vi "Set LCD to first pixel.vi"(8 "error in":errorcluster, 11 "FPGA VI Reference In":T1) -> (0 "error out":errorcluster, 3 "FPGA VI Reference Out":T1)   [LabVIEW 2019]
uses:
  TypeDefs/FPGA Reference.ctl
  <vilib>/Utility/error.llb/Error Cluster From Error Code.vi
  <vilib>/rvi/errors/niLvFpgaAdjustHostInterfaceError.vi
  <vilib>/rvi/interface/nirviReadWriteControl/nirviReadWriteControl.xnode
  FPGA Bitfiles/adafruitlcdsom_FPGATarget_FPGAMain_K7l+4zj6vFY.lvbitx
  FPGA Main.vi
  NiFpgaLv.dll
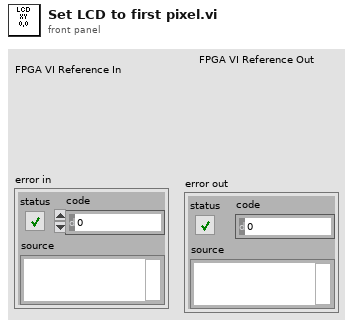
[diagram p1: front panel]
types:
  T1 = typedef "FPGA Reference.ctl" = refnum<k20>
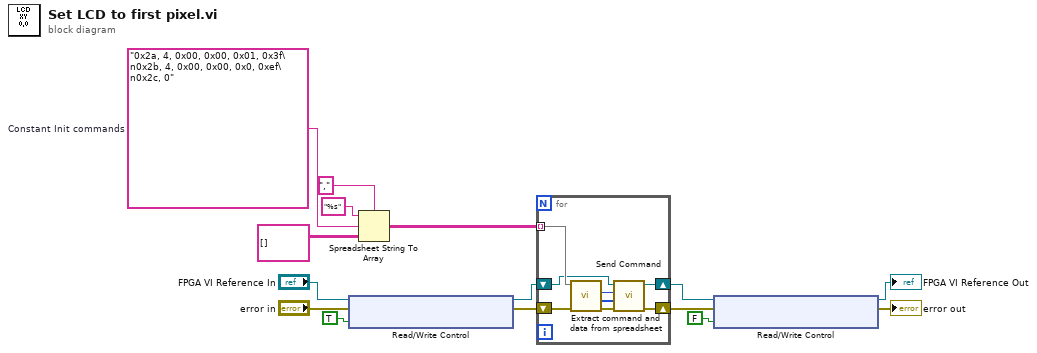
[diagram p0: block diagram]
diagram:
  w3 = "0x2a, 4, 0x00, 0x00, 0x01, 0x3f\n0x2b, 4, 0x00, 0x00, 0x0, 0xef\n0x2c, 0"  # Constant Init commands
  n1 = xnode "Read/Write Control"("FPGA VI Reference In"="FPGA VI Reference In", "error in"="error in", "StreamDisabled"=TRUE) -> ("FPGA VI Reference Out"=w9:T1, "error out"=w8:errorcluster)
  n2 = Spreadsheet String To Array(delimiter (Tab)=",", format string="%s", spreadsheet string=w3, array type (2D Dbl)=string[][] []) -> (array=w12:string[][])
  n3 = for {
    tunnel: w12 -> [w23] mode=indexing
    shift-right: [w21] -> w5
    shift-left: w8 -> [w19]
    shift-right: [w22] -> w4
    shift-left: w9 -> [w20]
    n4 = call "Extract command and data from spreadsheet.vi"("error in"=w19, "Data spreadsheet"=w23) -> ("error out"=w16:errorcluster, "Data"=w17:u32[], "Command"=w18:u32)  [unwired: 7 in]
    n5 = call "Send Command.vi"("error in"=w16, "Data"=w17, "Command"=w18, "FPGA VI Reference In"=w20) -> ("error out"=w21:errorcluster, "FPGA VI Reference Out"=w22:T1)  [unwired: 6 in]
  }
  n6 = xnode "Read/Write Control"("FPGA VI Reference In"=w4, "error in"=w5, "StreamDisabled"=FALSE) -> ("FPGA VI Reference Out"=→"FPGA VI Reference Out":T1, "error out"=→"error out":errorcluster)
